vi "Demo5-Control_Panel.vi"() -> ()   [LabVIEW 2020]
panel:
  out "Settable Device Keywords":string[](array[string])
  out "Live Readback Values":string[](array[string])
  in  "Set All":bool
  in  "Set Values\n(Fully empty cells will not be set)":string[](array[string])
  out "Diode Trace":waveform(dbl)[](graph)
  out "Live Responses":string[](array[string])
  out "Non-Settable Device Keywords":string[](array[string])
  in  "IP Address of Remote Device":string="196.254.31.200"
  in  "Disconnect":bool
  # "Diode Demo - Display ADC Trace"
  # "Demonstrates display of the ADC trace, with background and signal regions masked, for the STM32 Diode Device."
  # "VI Instructions\n\n1. Make sure you know the Device IP Address.\n2. From Windows command prompt, confirm ping to IP address.\n3. Type the correct device IP address into this VI.\n3. Run this VI. *Note:* Only one TCP connection to the device's SCPI-like server can run at a time.\n4. When finished, disconnect safely from the device via the \"Disconnect\" toggle button. (Not the Abort button).\n\nCreated by Scott Feister on July 13, 2022."
  # "Settings *ARE NOT SAVED TO DEVICE* and are lost on device reset! Write them down!"
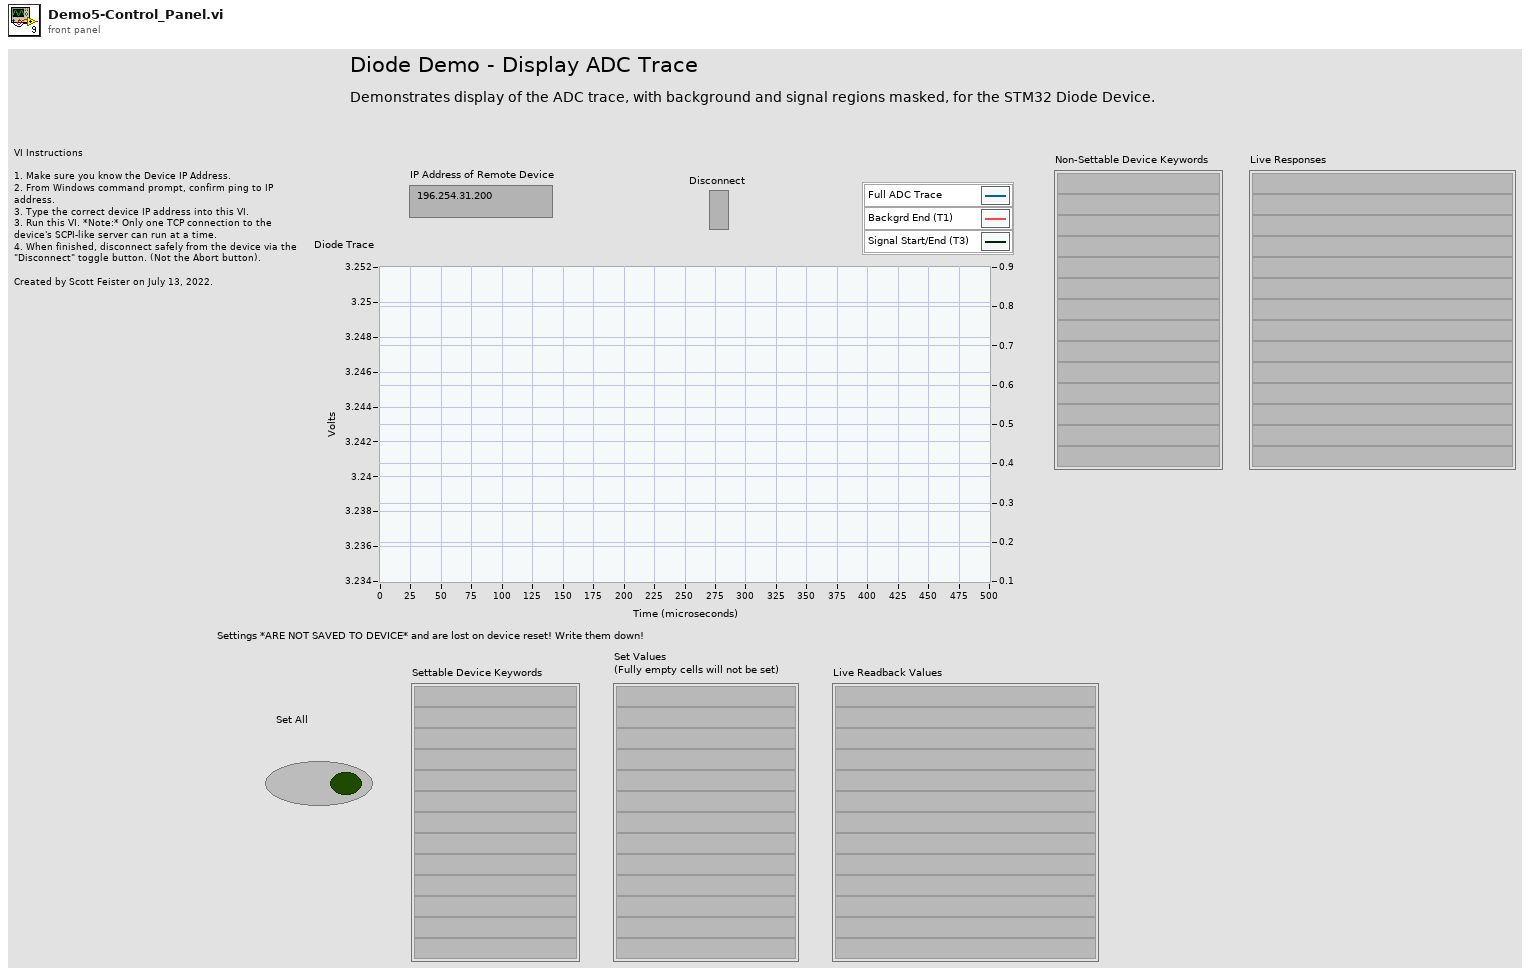
[diagram p1: front panel]
types:
  T1 = typedef "DDAQ-Keyword.ctl" = cluster{"Keyword":string, "Gettable":bool, "Settable":bool, "Is Array":bool, "Data Type":string, "Description":string}
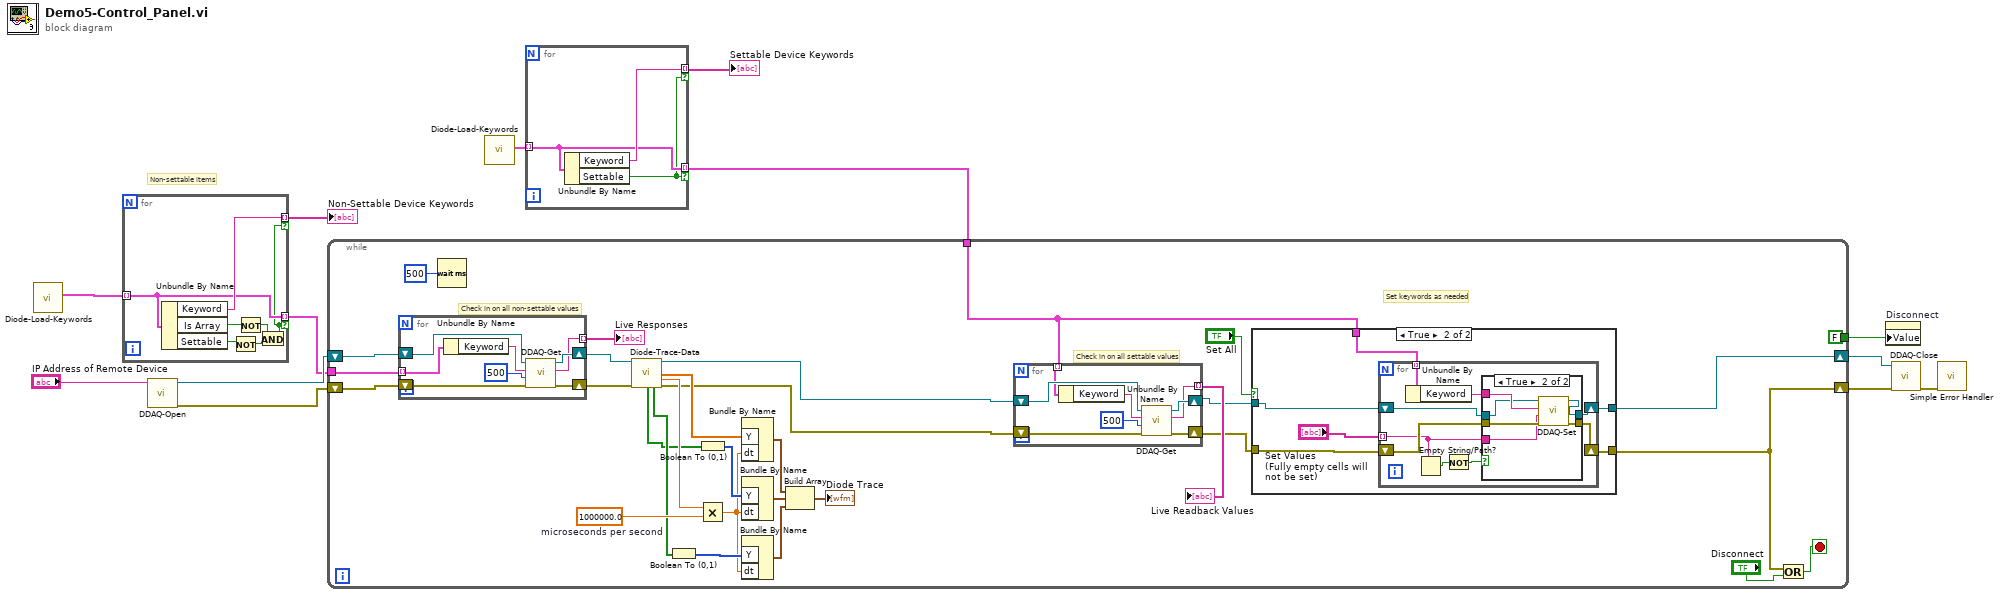
[diagram p0: block diagram]
diagram:
  # "Non-settable items"
  n1 = call "Diode-Load-Keywords.vi"() -> ("Diodes Keywords Array"=w6:T1[])  [unwired: 11 in]
  n2 = for {
    tunnel: w6 -> [w18] mode=indexing
    tunnel: [w20] -> w5 mode=indexing if=w14
    tunnel: [w18] -> w4 mode=indexing if=w14
    n3 = Unbundle By Name(w18) -> ("Keyword"=w20:string, "Is Array"=w19:bool, "Settable"=w17:bool)
    n4 = Not(x=w17) -> (.not. x?=w16:bool)
    n5 = Not(x=w19) -> (.not. x?=w15:bool)
    n6 = And(x=w15, y=w16) -> (x .and. y?=w14:bool)
  }
  "Non-Settable Device Keywords" <- w5
  n7 = call "DDAQ-Open.vi"("IP Address of Nucleo Device"="IP Address of Remote Device") -> ("error out"=w12:errorcluster, "connection ID"=w13:refnum<k5>)  [unwired: 8 in, 1 out]
  n8 = call "Diode-Load-Keywords.vi"() -> ("Diodes Keywords Array"=w3:T1[])  [unwired: 11 in]
  n9 = for {
    tunnel: w3 -> [w22] mode=indexing
    tunnel: [w23] -> w2 mode=indexing if=w21
    tunnel: [w22] -> w1 mode=indexing if=w21
    n10 = Unbundle By Name(w22) -> ("Keyword"=w23:string, "Settable"=w21:bool)
  }
  "Settable Device Keywords" <- w2
  n11 = while {
    shift-right: [w25] -> w11
    shift-left: w13 -> [w54]
    shift-right: [w24] -> w10
    shift-left: w12 -> [w53]
    tunnel: [FALSE] -> w8
    tunnel: w4 -> [w47]
    tunnel: w1 -> [w28]
    stop <- w49 stop-if-true
    w42 = 1000000.0  # microseconds per second
    # "Set keywords as needed"
    # "Check in on all settable values"
    # "Check in on all non-settable values"
    n12 = for {
      shift-right: [w93] -> w46
      shift-left: w54 -> [w95]
      shift-right: [w92] -> w45
      shift-left: w53 -> [w94]
      tunnel: [w90] -> w48 mode=indexing
      tunnel: w47 -> [w89] mode=indexing
      n13 = Unbundle By Name(w89) -> ("Keyword"=w88:string)
      n14 = call "DDAQ-Get.vi"("error in (no error)"=w94, "max bytes to read (10000)"=500 ("max bytes to read (500)"), "SCPI-like Keyword (leave off question mark)"=w88, "connection ID"=w95) -> ("error out"=w92:errorcluster, "Response"=w90:string, "connection ID out"=w93:refnum<k5>)  [unwired: 3 in, 2 out]
    }
    "Live Responses" <- w48
    n15 = Wait (ms)(milliseconds to wait=u32 500) -> ()  [unwired: 1 out]
    n16 = call "Diode-Trace-Data.vi"("connection ID"=w46, "error in (no error)"=w45) -> ("connection ID out"=w27:refnum<k5>, "Trace (Volts)"=w44:dbl[], "dt"=w43:dbl, "Background Mask Array"=w33:bool[], "Signal Mask Array"=w34:bool[], "error out"=w26:errorcluster)  [unwired: 5 in, 3 out]
    n17 = Boolean To (0,1)(Boolean=w34) -> (0, 1=w40:i16[])
    n18 = Boolean To (0,1)(Boolean=w33) -> (0, 1=w41:i16[])
    n19 = Multiply(x=w43, y=w42) -> (x*y=w39:dbl)
    n20 = Bundle By Name("Y"=w44, "dt"=w39) -> (w36:waveform(dbl))  [unwired: 1 in]
    n21 = Bundle By Name("Y"=w41, "dt"=w39) -> (w38:waveform(i16))  [unwired: 1 in]
    n22 = Bundle By Name("Y"=w40, "dt"=w39) -> (w37:waveform(i16))  [unwired: 1 in]
    n23 = Build Array(w36, w38, w37) -> (→"Diode Trace":waveform(dbl)[])
    n24 = for {
      shift-right: [w85] -> w30
      shift-left: w27 -> [w87]
      shift-right: [w84] -> w29
      shift-left: w26 -> [w86]
      tunnel: [w82] -> w32 mode=indexing
      tunnel: w28 -> [w81] mode=indexing
      n25 = Unbundle By Name(w81) -> ("Keyword"=w80:string)
      n26 = call "DDAQ-Get.vi"("error in (no error)"=w86, "max bytes to read (10000)"=500 ("max bytes to read (500)"), "SCPI-like Keyword (leave off question mark)"=w80, "connection ID"=w87) -> ("error out"=w84:errorcluster, "Response"=w82:string, "connection ID out"=w85:refnum<k5>)  [unwired: 3 in, 2 out]
    }
    "Live Readback Values" <- w32
    n27 = case shown="True" "Set All" {
      tunnel: w28 -> [_ w61]
      tunnel: w30 -> [w55 w60]
      tunnel: w29 -> [w56 w59]
      tunnel: [w56 w58] -> w24
      tunnel: [w55 w57] -> w25
      frame False {
      }
      frame True {
        n28 = for {
          tunnel: "Set Values\n(Fully empty cells will not be set)" -> [w63] mode=indexing
          tunnel: w61 -> [w71] mode=indexing
          shift-right: [w65] -> w58
          shift-left: w59 -> [w66]
          shift-right: [w64] -> w57
          shift-left: w60 -> [w69]
          n29 = Unbundle By Name(w71) -> ("Keyword"=w70:string)
          n30 = Empty String/Path?(string/path=w63) -> (empty?=w67:bool)
          n31 = Not(x=w67) -> (.not. x?=w68:bool)
          n32 = case shown="True" w68 {
            tunnel: w70 -> [_ w79]
            tunnel: w69 -> [w72 w78]
            tunnel: w66 -> [w73 w77]
            tunnel: [w73 w76] -> w65
            tunnel: [w72 w75] -> w64
            tunnel: w63 -> [_ w74]
            frame False {
            }
            frame True {
              n33 = call "DDAQ-Set.vi"("error in (no error)"=w77, "Set Value"=w74, "SCPI-like Keyword (leave off space, value)"=w79, "connection ID"=w78) -> ("error out"=w76:errorcluster, "connection ID out"=w75:refnum<k5>)  [unwired: 5 in, 1 out]
            }
          }
        }
      }
    }
    n34 = Or(x=w24, y="Disconnect") -> (x .or. y?=w49:bool)
  }
  n35 = property on="Disconnect" class="Bool (strict)"("Value"=w8) -> ()  [unwired: 2 in, 2 out]
  n36 = call "DDAQ-Close.vi"("error in (no error)"=w10, "connection ID"=w11) -> ("error out"=w9:errorcluster)  [unwired: 8 in, 1 out]
  n37 = call <vilib>:"Simple Error Handler.vi"("error in (no error)"=w9) -> ()  [unwired: 4 in, 5 out]
